vi "main.vi"() -> ()   [LabVIEW 2015]
uses:
  Typedefs/TestScenarioTypes.ctl
  Typedefs/TestExecution.ctl
  Model/TestScenarioFactory/TestScenarioFactory/TestScenarioFactory.lvclass
  Model/TestLogFactory/TestLogFactory/TestLogFactory.lvclass
  Typedefs/TestLogTypes.ctl
  Model/TestLog/ITestLog/ITestLog.lvclass
  Model/TestScenario/ITestScenario/ITestScenario.lvclass
  Typedefs/ILCBTTypedefs.lvlib
  <userlib>/Common/ILC/ILC/ILC.lvclass
panel:
  in  "End Testing":bool
  in  "Begin Testing":bool
  out "error out":errorcluster
  out "Result":T1
  in  "Serial Number":string
  in  "Stop":bool
  in  "Execute":bool
  in  "Test Scenario":T2
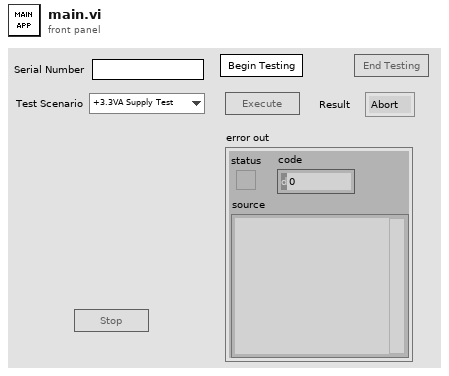
[diagram p1: front panel]
types:
  T1 = typedef "ILCBTTypedefs.lvlib/TestExecution.ctl" = enum16{"Abort", "Continue"}
  T2 = typedef "ILCBTTypedefs.lvlib/TestScenarioTypes.ctl" = enum16{"+3.3VA Supply Test", "+3.3VD Supply Test", "+5VA Supply Test", "+5VD Supply Test", "Unique ID Test", "TEDS Status Test", "LIMSW1_TTL Low Test", "LIMSW1_TTL High Test", "LIMSW2_TTL Low Test", "LIMSW2_TTL High Test", "Tachometer Test", "SSR_TTL Low Test", "SSR_TTL High Test", "SM_CW Low Test", "SM_CW High Test", "SM_CCW Low Test", "SM_CCW High Test", "SM_GPI Low Test", "SM_GPI High Test", "CW Motion Without Limit Test", "CW Motion With Limit Test", "CW Motion With Limit Interruption Test", "CW Motion on CCW Limit Test", "CCW Motion Without Limit Test", "CCW Motion With Limit Test", "CCW Motion With Limit Interruption Test", "CCW Motion on CW Limit Test", "RS232-TXD Low Test", "RS232-TXD High Test", "RS232-RTS Low Test", "RS232-RTS High Test", "RS232-RXD Low Test", "RS232-RXD High Test", "RS232-CTS Low Test", "RS232-CTS High Test", "Out_SS Low Test", "Out_SS High Test", "Out_SDI Low Test", "Out_SDI High Test", "Out_SCLK Low Test", "Out_SCLK High Test", "Reset Low Test", "Reset High Test", "1 Channel ADC Test", "3 Channel ADC Test", "5 Channel ADC Test", "Vref Test", "ROT Test", "DAC1 Test", "DAC2 Test", "DAC3 Test", "DAC4 Test", "BIAS Test", "EXC1 Test", "EXC2 Test", "EXC3 Test", "EXC4 Test"}
  T3 = enum8{"Enabled", "Disabled", "Disabled and Grayed Out"}
  T4 = typedef "ILCBTTypedefs.lvlib/ILC Settings.ctl" = cluster{"Supply Voltage Tests":T5, "Device Configuration Tests":T7, "ILC Digital Input Tests":T9, "ILC Digital Output Tests":T13, "ILC Analog Output Tests":T20, "ILC Analog Input Tests":T25, "Collection Settings":T29}
  T5 = typedef "ILCBTTypedefs.lvlib/Supply Voltage Tests.ctl" = cluster{"3.3 V Supply":T6, "5 V Supply":T6}
  T6 = typedef "ILCBTTypedefs.lvlib/Supply Voltage Test.ctl" = cluster{"Analog Supply DAQ Channel to Read":refnum<k21>, "Digital Supply DAQ Channel to Read":refnum<k21>, "Expected Value":dbl[unit], "Tolerance":dbl[unit]}
  T7 = typedef "ILCBTTypedefs.lvlib/Device Configuration Tests.ctl" = cluster{"TEDS Status Test":T8}
  T8 = typedef "ILCBTTypedefs.lvlib/1-Wire Test.ctl" = cluster{"Expected Value":string}
  T9 = typedef "ILCBTTypedefs.lvlib/ILC Digital Input Tests.ctl" = cluster{"Limit Switch 1:":T10, "Limit Switch 2:":T10, "General Purpose Digital Input":T11}
  T10 = typedef "ILCBTTypedefs.lvlib/ILC Digital Input Test.ctl" = cluster{"DAQmx Global Channel":refnum<k21>, "High Level Value to Test":enum16{"Low", "High"}, "High Level Value to Expect":enum16{"Low", "High"}, "Low Level Value to Test":enum16{"Low", "High"}, "Low Level Value to Expect":enum16{"Low", "High"}}
  T11 = typedef "ILCBTTypedefs.lvlib/ILC GPI Digital Input Test.ctl" = cluster{"DAQ Channel to Write":refnum<k21>, "Frequency Values to Test":T12}
  T12 = typedef "ILCBTTypedefs.lvlib/Test Values.ctl" = cluster{"Start Value":dbl, "Stop Value":dbl, "Number of Steps":u16}
  T13 = typedef "ILCBTTypedefs.lvlib/ILC Digital Output Tests.ctl" = cluster{"SSR":T14, "UART Serial Test":T16, "SSI Serial Test":T18, "Motor Drive Test":T19}
  T14 = typedef "ILCBTTypedefs.lvlib/ILC Digital Output Test.ctl" = cluster{"DAQ Channel to Read":refnum<k21>, "High Level Value to Test":T15, "High Level Value to Expect":T15, "Low Level Value to Test":T15, "Low Level Value to Expect":T15}
  T15 = typedef "ILCBTTypedefs.lvlib/Digital Signal Level.ctl" = enum16{"Low", "High"}
  T16 = typedef "ILCBTTypedefs.lvlib/UART Serial Test.ctl" = cluster{"MUX Settings":T17, "CTS":T14, "TXD":T14, "RTS":T14, "RXD":T14}
  T17 = typedef "ILCBTTypedefs.lvlib/MUX Settings.ctl" = cluster{"MUX_AO":T15, "MUX_A1":T15, "MUX_A0 DAQ Channel to Write":refnum<k21>, "MUX_A1 DAQ Channel to Write":refnum<k21>}
  T18 = typedef "ILCBTTypedefs.lvlib/SSI Serial Test.ctl" = cluster{"MUX Settings":T17, "Out_SS":T14, "Out_SDI":T14, "Out_SCLK":T14, "Reset":T14}
  T19 = typedef "ILCBTTypedefs.lvlib/Motor Drive Test.ctl" = cluster{"MUX Settings":T17, "SM_CW":T14, "SM_CCW":T14, "SM_GPI":T14}
  T20 = typedef "ILCBTTypedefs.lvlib/ILC Analog Output Tests.ctl" = cluster{"Delay Between Test Steps":u16, "Vref":T21, "ROT":T22, "BIAS":T21, "EXC":T23, "DAC":T24}
  T21 = typedef "ILCBTTypedefs.lvlib/ILC Static Analog Output Test.ctl" = cluster{"DAQ Channel to Read":refnum<k21>, "Expected Value":dbl[unit], "Tolerance":dbl[unit]}
  T22 = typedef "ILCBTTypedefs.lvlib/ILC Analog Output Test.ctl" = cluster{"DAQ Channel to Read":refnum<k21>, "Test Values":T12, "Tolerance":dbl[unit]}
  T23 = typedef "ILCBTTypedefs.lvlib/ILC EXC Analog Output Test.ctl" = cluster{"EXC1 DAQ Channel to Read":refnum<k21>, "EXC2 DAQ Channel to Read":refnum<k21>, "EXC3 DAQ Channel to Read":refnum<k21>, "EXC4 DAQ Channel to Read":refnum<k21>, "Expected Value":dbl[unit], "Tolerance":dbl[unit]}
  T24 = typedef "ILCBTTypedefs.lvlib/ILC DAC Analog Output Test.ctl" = cluster{"DAC1 DAQ Channel to Read":refnum<k21>, "DAC2 DAQ Channel to Read":refnum<k21>, "DAC3 DAQ Channel to Read":refnum<k21>, "DAC4 DAQ Channel to Read":refnum<k21>, "Test Values":T12, "Tolerance":dbl[unit]}
  T25 = typedef "ILCBTTypedefs.lvlib/ILC Analog Input Tests.ctl" = cluster{"CH13 DAQ Channel to Write":refnum<k21>, "CH24 DAQ Channel to Write":refnum<k21>, "AO Voltage Data":T26, "Delay Between Test Steps":u16, "1 Channel":T27, "3 Channels":T28, "5 Channels":T28}
  T26 = typedef "ILCBTTypedefs.lvlib/AI Voltage to NI Voltage.ctl" = cluster{"ADC Bit Count":u16, "Vref":dbl[unit], "NI Scaling":dbl, "Bias":dbl[unit]}
  T27 = typedef "ILCBTTypedefs.lvlib/ILC Ch0 Analog Input Test.ctl" = cluster{"ADC Configurations":string[], "Value to Expect":i32, "Tolerance":i32, "PGA Gain Coefficients":u16[]}
  T28 = typedef "ILCBTTypedefs.lvlib/Multichannel Analog Input Test.ctl" = cluster{"ADC Configurations":string[], "PGA Gain Coefficients":u16[], "Test Values":T12, "Tolerance":dbl[unit]}
  T29 = typedef "ILCBTTypedefs.lvlib/Collection Settings.ctl" = cluster{"Samples To Average":u32}
  T30 = typedef "ILCBTTypedefs.lvlib/TestLogTypes.ctl" = enum16{"CSV Test Log"}
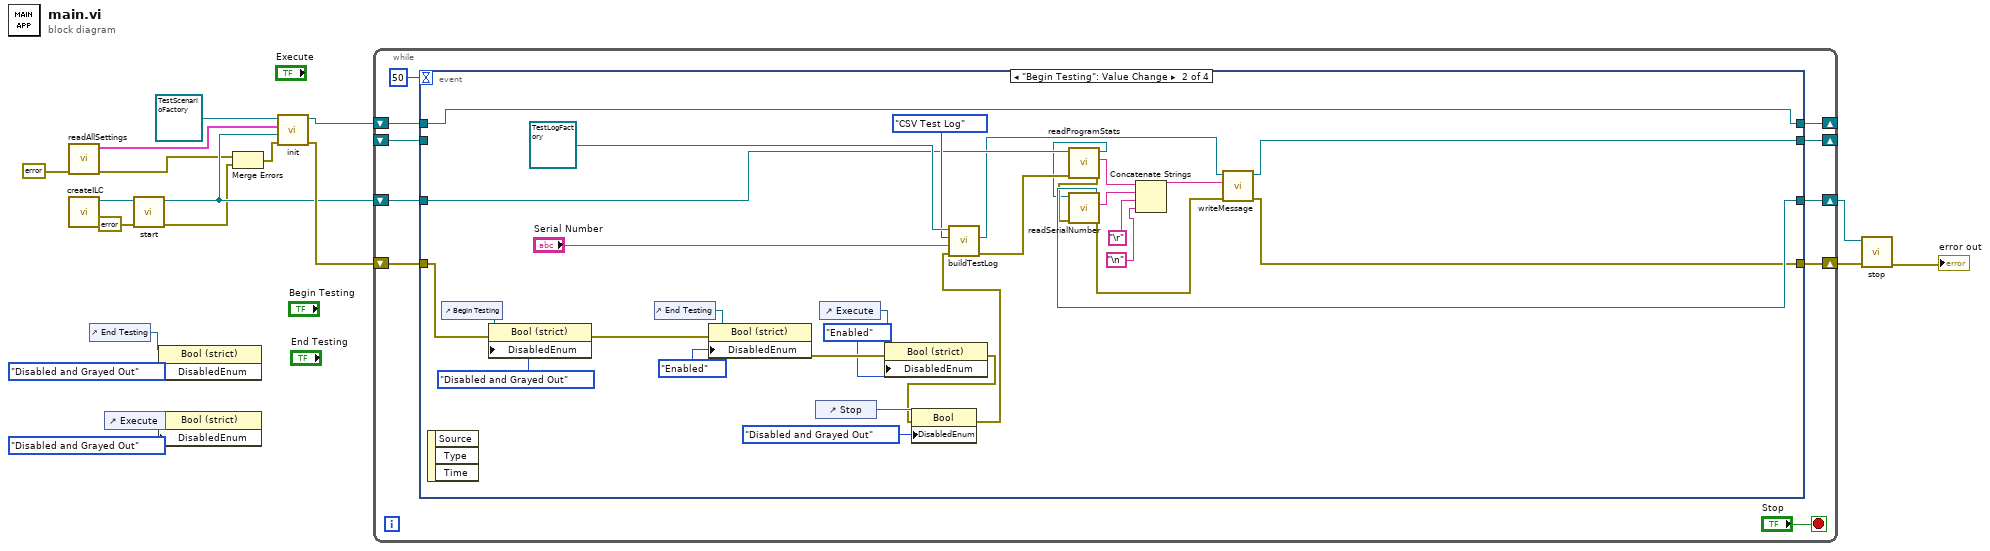
[diagram p0: block diagram]
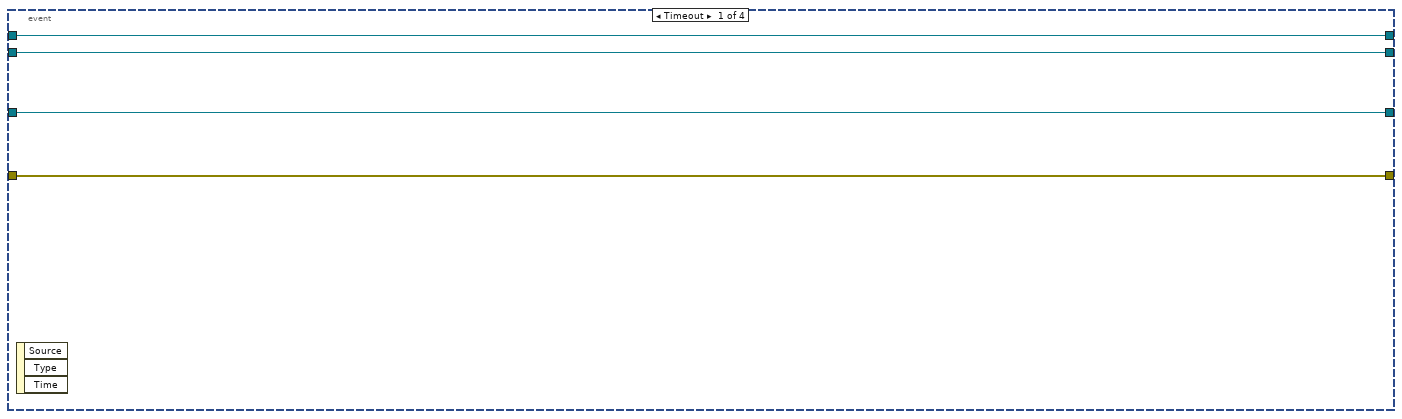
[diagram p2: hidden frame]
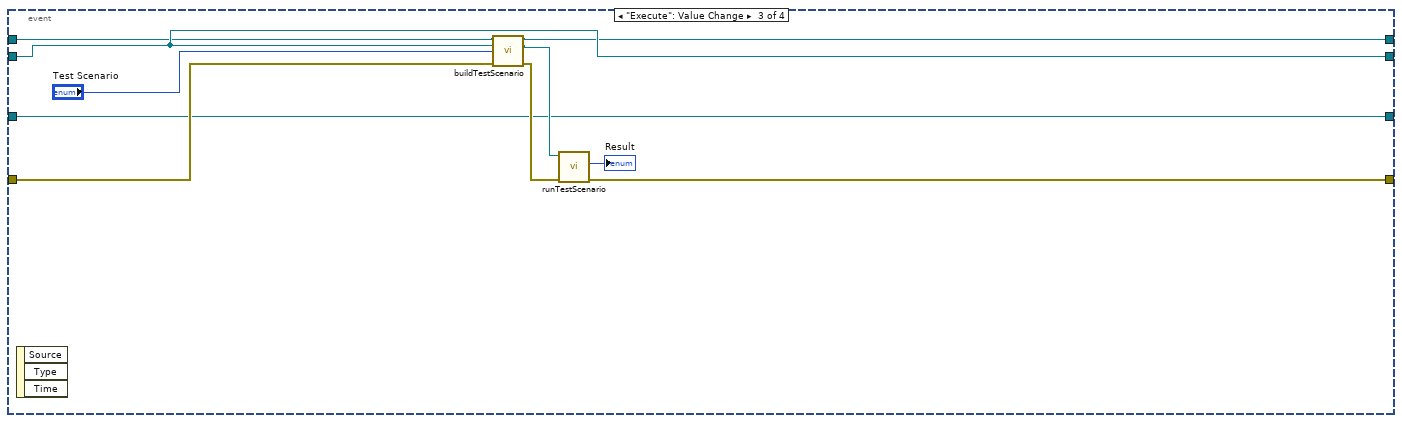
[diagram p3: hidden frame]
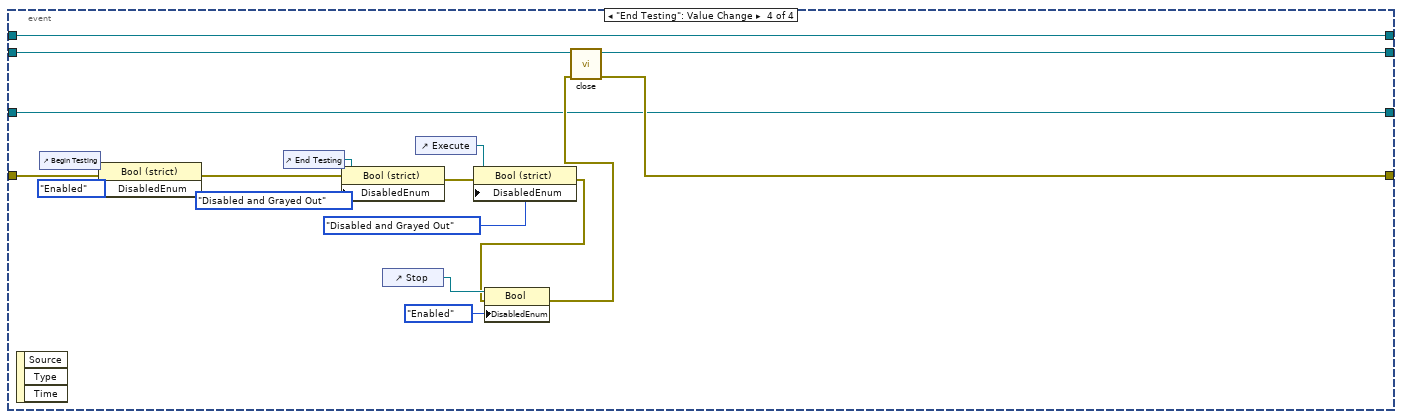
[diagram p4: hidden frame]
diagram:
  n1 = call "readAllSettings.vi"("error in (no error)"=errorcluster {"status"=FALSE, "code"=0, "source"=""}) -> ("error out"=w5:errorcluster, "ILC Settings"=w9:T4)  [unwired: 9 in]
  n2 = call "createILC.vi"() -> ("ILC"=w11:refnum<class "ILC.lvclass">)  [unwired: 11 in]
  n3 = control-ref of="End Testing"() -> (w18:refnum<vi>)
  n4 = control-ref of="Execute"() -> (w16:refnum<vi>)
  n5 = call <userlib>:"start.vi"("error in (no error)"=errorcluster {"status"=FALSE, "code"=0, "source"=""}, "ILC in"=w11) -> ("error out"=w6:errorcluster, "ILC out"=w8:refnum<class "ILC.lvclass">)  [unwired: 8 in]
  n6 = property class="Bool (strict)"(reference=w18, "DisabledEnum"=T3."Disabled and Grayed Out" ("Disabled")) -> ()  [unwired: 1 in, 2 out]
  n7 = property class="Bool (strict)"(reference=w16, "DisabledEnum"=T3."Disabled and Grayed Out" ("Disabled")) -> ()  [unwired: 1 in, 2 out]
  n8 = Merge Errors(w5, w6) -> (w7:errorcluster)
  n9 = call-dynamic "init.vi"("error in (no error)"=w7, "ILC"=w8, "ILC Settings"=w9, "TestScenarioFactory in"=refnum<class "TestScenarioFactory.lvclass"> refnum ("TestScenarioFactory.lvclass")) -> ("error out"=w12:errorcluster, "TestScenarioFactory out"=w13:refnum<class "TestScenarioFactory.lvclass">)  [unwired: 6 in]
  n10 = while {
    shift-right: [w25] -> _
    shift-left: w13 -> [w26]
    shift-right: [w24] -> w3
    shift-left: w12 -> [w23]
    shift-right: [w22] -> _
    shift-left: _ -> [w21]
    shift-right: [w19] -> w1
    shift-left: w8 -> [w20]
    stop <- "Stop" stop-if-true
    n11 = event shown="[1] \"Begin Testing\": Value Change" {
      selector: _ -> [_ _ _ _]
      dyn-events: _ -> [_ _ _ _]
      timeout: 50 -> [_ _ _ _]
      tunnel: w26 -> [w32 w60 w67 w91]
      tunnel: [w32 w60 w66 w91] -> w25
      tunnel: [w31 w37 w72 w84] -> w24
      tunnel: w23 -> [w31 w51 w70 w87]
      tunnel: [w30 w35 w68 w89] -> w22
      tunnel: w21 -> [w30 _ w68 w90]
      tunnel: w20 -> [w29 w44 w64 w74]
      tunnel: [w29 w43 w64 w74] -> w19
      event Timeout {
        n12 = event-data() -> ()  [unwired: 1 in, 3 out]
      }
      event "Begin Testing": Value Change {
        n13 = event-data() -> ()  [unwired: 1 in, 3 out]
        n14 = control-ref of="Begin Testing"() -> (w58:refnum<vi>)
        n15 = property class="Bool (strict)"(reference=w58, error in=w51, "DisabledEnum"=T3."Disabled and Grayed Out" ("Disabled")) -> (error out=w59:errorcluster)  [unwired: 1 out]
        n16 = control-ref of="End Testing"() -> (w56:refnum<vi>)
        n17 = property class="Bool (strict)"(reference=w56, error in=w59, "DisabledEnum"=T3."Enabled" ("Disabled")) -> (error out=w53:errorcluster)  [unwired: 1 out]
        n18 = control-ref of="Stop"() -> (w50:refnum<vi>)
        n19 = control-ref of="Execute"() -> (w54:refnum<vi>)
        n20 = property class="Bool (strict)"(reference=w54, error in=w53, "DisabledEnum"=T3."Enabled" ("Disabled")) -> (error out=w48:errorcluster)  [unwired: 1 out]
        n21 = property class="Bool"(reference=w50, error in=w48, "DisabledEnum"=T3."Disabled and Grayed Out" ("Disabled")) -> (error out=w47:errorcluster)  [unwired: 1 out]
        n22 = call-dynamic "buildTestLog.vi"("error in (no error)"=w47, "Serial Number"="Serial Number", "TestLogTypes"=TestLogTypes."CSV Test Log", "TestLogFactory in"=refnum<class "TestLogFactory.lvclass"> refnum ("TestLogFactory.lvclass")) -> ("error out"=w42:errorcluster, "ITestLog.lvclass"=w36:refnum<class "ITestLog.lvclass">)  [unwired: 5 in, 1 out]
        n23 = call <userlib>:"readProgramStats.vi"("error in (no error)"=w42, "ILC in"=w44) -> ("error out"=w41:errorcluster, "Response"=w46:string, "ILC out"=w40:refnum<class "ILC.lvclass">)  [unwired: 7 in]
        n24 = call <userlib>:"readSerialNumber.vi"("error in (no error)"=w41, "ILC in"=w40) -> ("error out"=w38:errorcluster, "Serial Number"=w45:string, "ILC out"=w43:refnum<class "ILC.lvclass">)  [unwired: 7 in]
        n25 = Concatenate Strings(w46, w45, "\r", "\n") -> (w39:string)
        n26 = call-dynamic "writeMessage.vi"("error in (no error)"=w38, "Message"=w39, "ITestLog in"=w36) -> ("error out"=w37:errorcluster, "ITestLog out"=w35:refnum<class "ITestLog.lvclass">)  [unwired: 7 in]
      }
      event "Execute": Value Change {
        n27 = event-data() -> ()  [unwired: 1 in, 3 out]
        n28 = call-dynamic "buildTestScenario.vi"("TestScenarioFactory in"=w67, "Log"=w68, "Test Scenario"="Test Scenario", "error in (no error)"=w70) -> ("TestScenarioFactory out"=w66:refnum<class "TestScenarioFactory.lvclass">, "ITestScenario.lvclass"=w65:refnum<class "ITestScenario.lvclass">, "error out"=w71:errorcluster)  [unwired: 9 in]
        n29 = call-dynamic "runTestScenario.vi"("error in (no error)"=w71, "ITestScenario in"=w65) -> ("error out"=w72:errorcluster, "TestExecution"=→"Result":T1)  [unwired: 7 in, 1 out]
      }
      event "End Testing": Value Change {
        n30 = event-data() -> ()  [unwired: 1 in, 3 out]
        n31 = control-ref of="Begin Testing"() -> (w88:refnum<vi>)
        n32 = property class="Bool (strict)"(reference=w88, error in=w87, "DisabledEnum"=T3."Enabled" ("Disabled")) -> (error out=w85:errorcluster)  [unwired: 1 out]
        n33 = control-ref of="End Testing"() -> (w82:refnum<vi>)
        n34 = property class="Bool (strict)"(reference=w82, error in=w85, "DisabledEnum"=T3."Disabled and Grayed Out" ("Disabled")) -> (error out=w80:errorcluster)  [unwired: 1 out]
        n35 = control-ref of="Stop"() -> (w78:refnum<vi>)
        n36 = control-ref of="Execute"() -> (w81:refnum<vi>)
        n37 = property class="Bool (strict)"(reference=w81, error in=w80, "DisabledEnum"=T3."Disabled and Grayed Out" ("Disabled")) -> (error out=w77:errorcluster)  [unwired: 1 out]
        n38 = property class="Bool"(reference=w78, error in=w77, "DisabledEnum"=T3."Enabled" ("Disabled")) -> (error out=w75:errorcluster)  [unwired: 1 out]
        n39 = call-dynamic "close.vi"("error in (no error)"=w75, "ITestLog in"=w90) -> ("error out"=w84:errorcluster, "ITestLog out"=w89:refnum<class "ITestLog.lvclass">)  [unwired: 8 in]
      }
    }
  }
  n40 = call <userlib>:"stop.vi"("error in (no error)"=w3, "ILC in"=w1) -> ("error out"=→"error out":errorcluster)  [unwired: 8 in, 1 out]
